vi "get_DSC.vi"(8 "error in (no error)":errorcluster, 11 "HGF_DSCSubscriber.lvclass in":refnum<class "HGF_DSCSubscriber.lvclass">) -> (0 "error out":errorcluster, 2 "Shared Variable":refnum<k21>, 3 "HGF_DSCSubscriber.lvclass out":refnum<class "HGF_DSCSubscriber.lvclass">)   [LabVIEW 2012, in "HGF_DSC.lvlib" / "HGF_DSCSubscriber.lvclass"]
uses:
  HGF_DSCSubscriber.lvclass
  HGF_DSCSubscriber.lvclass/HGF_DSCSubscriber.ctl
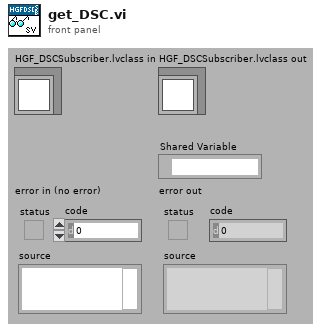
[diagram p1: front panel]
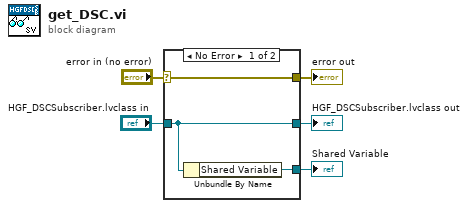
[diagram p0: block diagram]
diagram:
  n1 = case shown="No Error" "error in (no error)" {
    selector: "error in (no error)" -> [w8 w9]
    tunnel: [w8 w9] -> w4
    tunnel: [w7 w10] -> w2
    tunnel: "HGF_DSCSubscriber.lvclass in" -> [w7 w10]
    tunnel: [w6 _] -> w1
    frame No Error {
      n2 = Unbundle By Name(w7) -> ("Shared Variable"=w6:refnum<k21>)
    }
    frame Error {
    }
  }
  "error out" <- w4
  "HGF_DSCSubscriber.lvclass out" <- w2
  "Shared Variable" <- w1
